vi "CheckWriteReadError.vi"(1 "error":errorcluster, 2 "Subscriber in":T1, 3 "Connections in":T2(array[cluster])) -> (0 "Connections out":T2(array[cluster]))   [LabVIEW 2010]
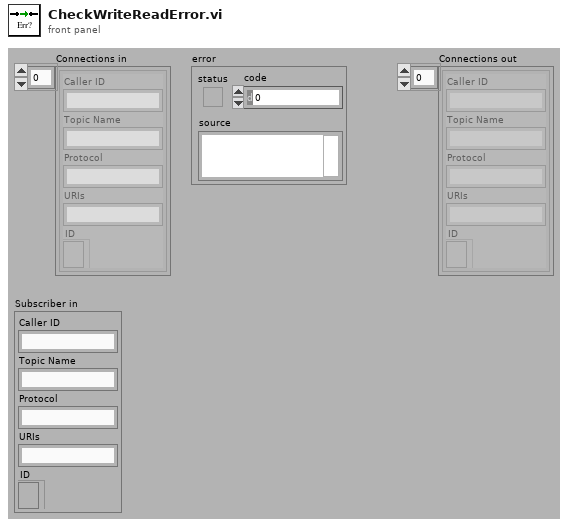
[diagram p1: front panel]
types:
  T1 = cluster{"Caller ID":string, "Topic Name":string, "Protocol":string, "URIs":string, "ID":refnum<k5>}
  T2 = cluster{"Caller ID":string, "Topic Name":string, "Protocol":string, "URIs":string, "ID":refnum<k5>}[]
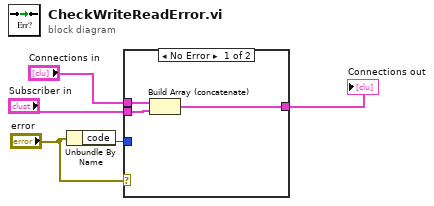
[diagram p0: block diagram]
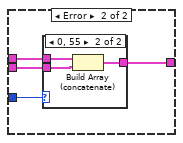
[diagram p2: hidden frame]
diagram:
  n1 = Unbundle By Name("error") -> ("code"=w2:i32)
  n2 = case shown="No Error" "error" {
    tunnel: "Subscriber in" -> [w7 w12]
    tunnel: w2 -> [_ w11]
    tunnel: [w6 w10] -> w4
    tunnel: "Connections in" -> [w8 w9]
    frame No Error {
      n3 = Build Array (concatenate)(w8, w7) -> (w6:T2)
    }
    frame Error {
      n4 = case shown="0, 55" w11 {
        tunnel: w12 -> [_ w16]
        tunnel: [w13 w15] -> w10
        tunnel: w9 -> [w13 w14]
        frame Default {
        }
        frame 0, 55 {
          n5 = Build Array (concatenate)(w14, w16) -> (w15:T2)
        }
      }
    }
  }
  "Connections out" <- w4
